vi "JSON to Palettes.vi"(11 "Material JSON":string) -> (0 "error out":errorcluster, 3 "Palettes":refnum<class "Material-Palette.lvclass">[](array[class]))   [LabVIEW 2021, in "TSC Material Theme.lvlib" / "Material-Palette.lvclass"]
doc: "read the json string of palette information and convert it into the array of classes for the theme\n\n<b>Code Developed By:</b> +\nDaniel Coons +\nTechnology Service Corporation +\nwww.tsc.com/atcs"
uses:
  Material-Palette.lvclass
  Serializer-Palette/Serializer-Palette.lvclass
  C:/Program Files/National Instruments/LabVIEW 2026/vi.lib/JDP Science/JSONtext/LVClass Serializer/JSONtext LVClass Serializer.lvclass
  Serializer-Palette/Serializer-Palette.lvclass/Serializer-Palette.ctl
  Material-Palette.lvclass/Material-Palette.ctl
  <vilib>/JDP Science/JSONtext/JSONtext.lvlib
  bcc1f051-5bb6-434e-b816-a57df783be2e.vi
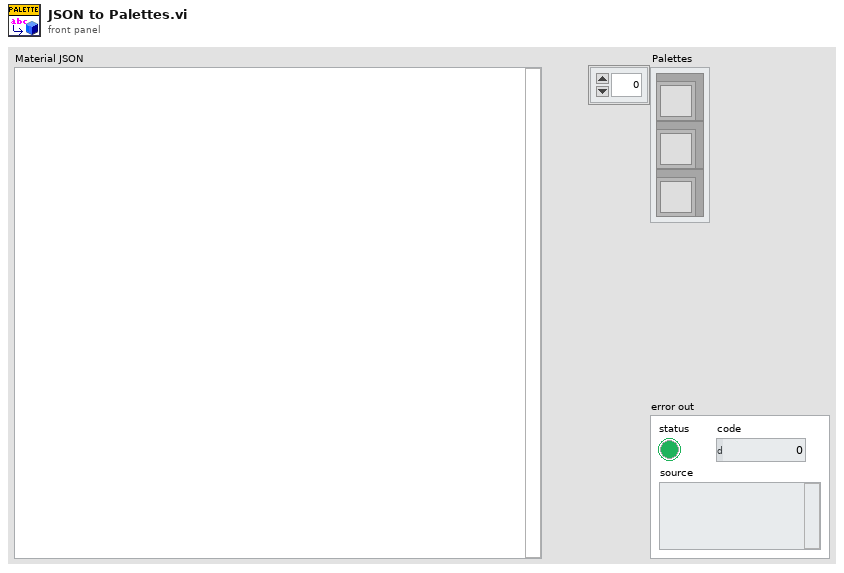
[diagram p1: front panel]
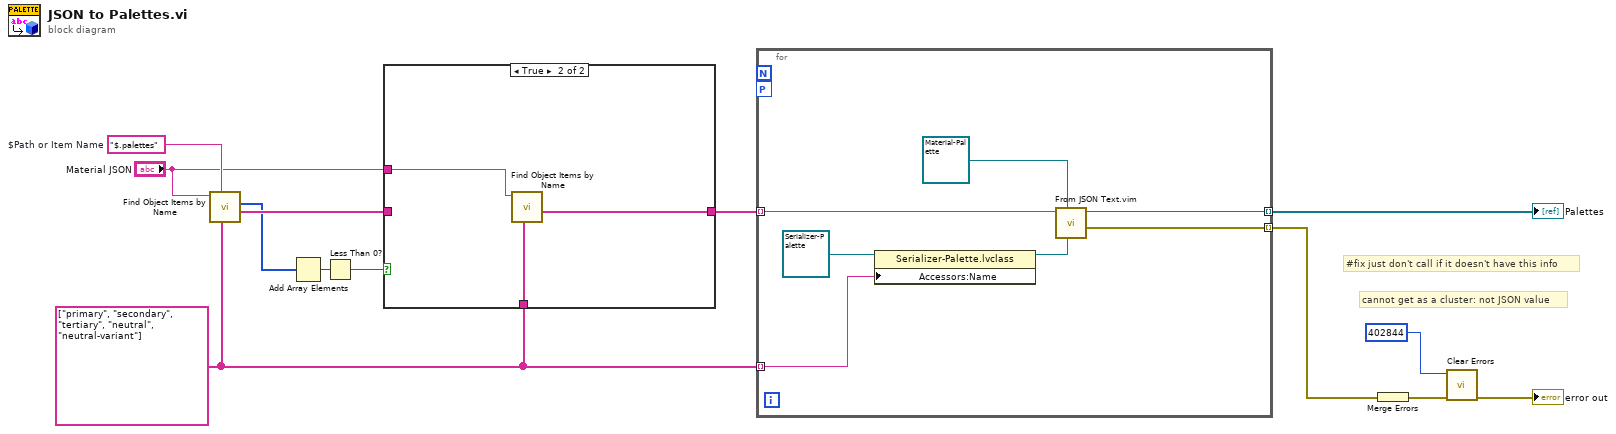
[diagram p0: block diagram]
diagram:
  w12 = "$.palettes"  # $Path or Item Name
  w8 = string[] ["primary", "secondary", "tertiary", "neutral", "neutral-variant"] ("Item Names")
  # "#fix just don't call if it doesn't have this info"
  # "cannot get as a cluster: not JSON value"
  n1 = call <vilib>:"Find Object Items by Name.vi"("Item Names"=w8, "$Path or Item Name"=w12, "JSON"="Material JSON") -> ("<JSON>"=w10:string[], "Offsets"=w6:i32[])  [unwired: 6 in, 1 out]
  n2 = Add Array Elements(numeric array=w6) -> (sum=w5:i32)
  n3 = Less Than 0?(x=w5) -> (x < 0?=w4:bool)
  n4 = case shown="True" w4 {
    tunnel: w10 -> [w14 _]
    tunnel: [w14 w15] -> w7
    tunnel: "Material JSON" -> [_ w17]
    tunnel: w8 -> [_ w16]
    frame False {
    }
    frame True {
      n5 = call <vilib>:"Find Object Items by Name.vi"("Item Names"=w16, "JSON"=w17) -> ("<JSON>"=w15:string[])  [unwired: 7 in, 2 out]
    }
  }
  n6 = for {
    tunnel: [w22] -> w11 mode=indexing
    tunnel: [w24] -> w13 mode=indexing
    tunnel: w7 -> [w21] mode=indexing
    tunnel: w8 -> [w18] mode=indexing
    workers-P: _ -> [_]
    n7 = property class="Serializer-Palette.lvclass"(reference=refnum<class "Serializer-Palette.lvclass"> refnum ("TSC Material Theme.lvlib:Serializer-Palette.lvclass"), "Accessors:Name"=w18) -> (reference out=w19:refnum<class "Serializer-Palette.lvclass">)  [unwired: 1 in, 1 out]
    n8 = call "From JSON Text.vim"("LVClass Serializer"=w19, "Data Type and Default Value"=refnum<class "Material-Palette.lvclass"> refnum ("TSC Material Theme.lvlib:Material-Palette.lvclass"), "JSON"=w21) -> ("error out"=w24:errorcluster, "Data out"=w22:refnum<class "Material-Palette.lvclass">)  [unwired: 7 in]
  }
  "Palettes" <- w11
  n9 = Merge Errors(w13) -> (w3:errorcluster)
  n10 = call <vilib>:"Clear Errors.vi"("error in (no error)"=w3, "specific error code to clear (0: all)"=402844) -> ("error out"=→"error out":errorcluster)  [unwired: 4 in, 1 out]
